vi "Zamojski_B_2.vi"   [LabVIEW 2020]
uses:
  <vilib>/Platform/TimedLoop/XDataNode/timing_clust.ctl
  <vilib>/Platform/TimedLoop/XDataNode/nitl_modes.ctl
  <vilib>/Platform/TimedLoop/XDataNode/wakeup.ctl
  <vilib>/platform/TimedLoop/XDataNode/XDataNode.xnode
  <vilib>/Platform/TimedLoop/XDataNode/XDNodeRunTimeDep.lvlib
types:
  T1 = typedef "Rendezvous RefNum" = refnum<k1>
  T2 = typedef "Semaphore RefNum" = refnum<k1>
  T3 = typedef "XDNodeRunTimeDep.lvlib/timing_clust.ctl" = cluster{"Expected End [f-1]":u64, "Actual End [f-1]":u64, "Finished Late? [f-1]":bool, "Expected End [i-1]":u64, "Actual End [i-1]":u64, "Finished Late? [i-1]":bool, "Expected Start [i]":u64, "Actual Start [i]":u64, "Expected Start [f]":u64, "Actual Start [f]":u64, "Source Name":string, "Structure Name":string, "Period":i64, "Deadline":i64, "Offset":i64, "Start":i64, "Priority":i32, "Timeout":i32, "Mode":T4, "Wakeup Reason":T5, "Error":errorcluster, "Source Type":string, "Secondary Source Type":string, "Global End Time":u64, "Global Start Time":u64, "Frame Duration":u64, "Iteration Duration":u64, "Assigned CPU":i32, "I/O Scan Engine Mode":u32}
  T4 = typedef "XDNodeRunTimeDep.lvlib/nitl_modes.ctl" = enum32{"No Change", "Process missed periods, maintain original phase", "Discard missed periods, maintain original phase", "Process missed periods, ignore original phase", "Discard missed periods, ignore original phase"}
  T5 = typedef "XDNodeRunTimeDep.lvlib/wakeup.ctl" = enum32{"Normal", "Aborted", "Asynchronous wakeup", "Timing source error", "Timed loop error", "Timeout"}
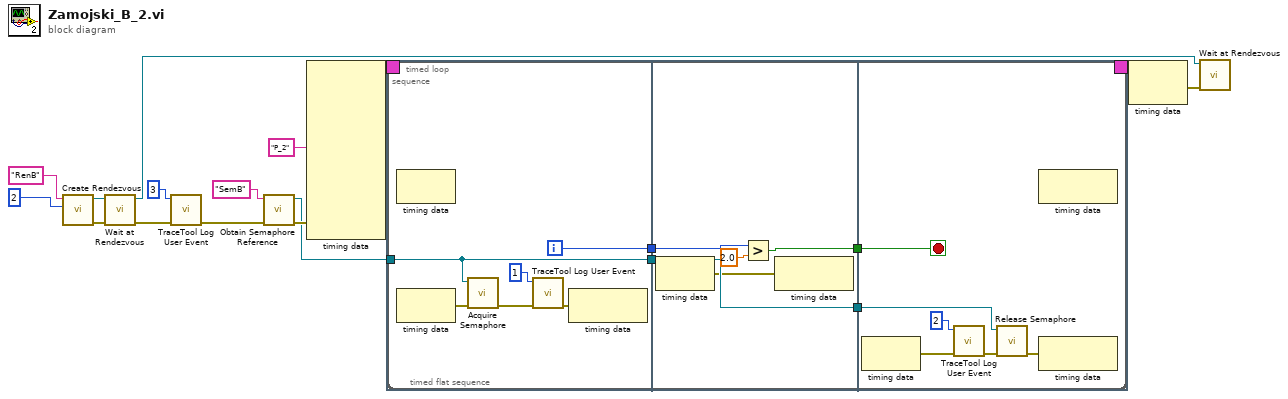
[diagram p0: block diagram]
diagram:
  n1 = call <vilib>:"Create Rendezvous.vi"("size (2)"=2, "name (unnamed)"="RenB") -> ("error out"=w12:errorcluster, "rendezvous"=w14:T1)  [unwired: 3 in, 1 out]
  n2 = call <vilib>:"Wait at Rendezvous.vi"("error in (no error)"=w12, "rendezvous"=w14) -> ("error out"=w11:errorcluster, "rendezvous out"=w2:T1)  [unwired: 3 in, 1 out]
  n3 = call <vilib>:"TraceTool Log User Event.vi"("error in (no error)"=w11, "Event ID (0-255)"=u32 3) -> ("error out"=w9:errorcluster)  [unwired: 9 in]
  n4 = call <vilib>:"Obtain Semaphore Reference.vi"("error in (no error)"=w9, "name (unnamed)"="SemB") -> ("error out"=w4:errorcluster, "semaphore"=w3:T2)  [unwired: 3 in, 1 out]
  n5 = node-c288("P_2" ("Structure Name"), w4) -> (w7:T3)  [unwired: 8 in]
  n6 = timed-loop {
    timing: w7 -> [_]
    timing-out: [_] -> w6
    tunnel: w3 -> [w16]
    i -> [w22]
    stop <- w43 stop-if-true
    n7 = timed-sequence {
      timing: _ -> [_]
      timing-out: _ -> [_]
      tunnel: w16 -> [w19]
      n8 = timed-flat-sequence {
        tunnel: [w23] -> w20
        tunnel: w19 -> [w23]
        tunnel: [w22] -> w18
        tunnel: [w37] -> w21
        tunnel: w20 -> [w37]
        tunnel: w18 -> [w35]
        tunnel: [w34] -> w17
        tunnel: w21 -> [w44]
        tunnel: w17 -> [w43]
        frame #0 {
          n9 = node-c288() -> (w27:errorcluster)  [unwired: 1 in]
          n10 = call <vilib>:"Acquire Semaphore.vi"("error in (no error)"=w27, "semaphore"=w23) -> ("error out"=w26:errorcluster)  [unwired: 3 in, 2 out]
          n11 = call <vilib>:"TraceTool Log User Event.vi"("error in (no error)"=w26, "Event ID (0-255)"=u32 1) -> ("error out"=w24:errorcluster)  [unwired: 9 in]
          n12 = node-c288(w24) -> ()  [unwired: 1 out]
        }
        frame #1 {
          n13 = node-c288() -> (w33:errorcluster)  [unwired: 1 in]
          n14 = Greater?(x=w35, y=2.0) -> (0:w34:bool)
          n15 = node-c288(w33) -> ()  [unwired: 1 out]
        }
        frame #2 {
          n16 = node-c288() -> (w47:errorcluster)  [unwired: 1 in]
          n17 = call <vilib>:"TraceTool Log User Event.vi"("error in (no error)"=w47, "Event ID (0-255)"=u32 2) -> ("error out"=w46:errorcluster)  [unwired: 9 in]
          n18 = call <vilib>:"Release Semaphore.vi"("error in (no error)"=w46, "semaphore"=w44) -> ("error out"=w45:errorcluster)  [unwired: 4 in, 1 out]
          n19 = node-c288(w45) -> ()  [unwired: 1 out]
        }
      }
    }
    n20 = node-c288() -> ()  [unwired: 1 in, 1 out]
    n21 = node-c288() -> ()  [unwired: 1 in, 1 out]
  }
  n22 = node-c288(w6) -> (w1:errorcluster)
  n23 = call <vilib>:"Wait at Rendezvous.vi"("error in (no error)"=w1, "rendezvous"=w2) -> ()  [unwired: 3 in, 3 out]
